vi "Send general mesage.vi"(4 "Content":variant, 6 "Topic":variant, 7 "Sender":string, 8 "error in (no error)":errorcluster, 9 "Recipient":string, 10 "Message":T1={"Sender"="", "Recipient"="", "Topic"=variant(string ""), "Content"=variant, "Time Stamp"=timestamp(0 s since 1904-01-01)} {"Time Stamp" format="%<%H:%M:%S\n%Y/%m/%d>T"}, 11 "Mailbox ref in":T2) -> (0 "error out":errorcluster, 2 "timed out?":bool, 3 "mailbox ref out":T2)   [LabVIEW 2021, in "MatS Libs.lvlib"]
doc: "Puts general message into mailbox. If any information is missing, it is autofilled with default value.\nDefault values:\nIf optional imputs are not empty, they obverwrites message cluster."
uses:
  <userlib>/MatS Libs/MatS Mailman/TypeDefs/Mailbox ref.ctl
  <userlib>/MatS Libs/MatS Mailman/TypeDefs/General message.ctl
  <userlib>/MatS Libs/MatS Libs.lvlib
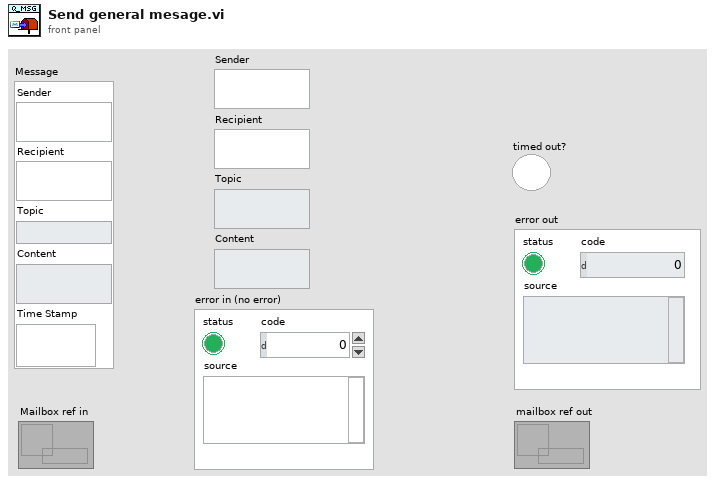
[diagram p1: front panel]
types:
  T1 = typedef "MatS Libs.lvlib/General message.ctl" = cluster{"Sender":string, "Recipient":string, "Topic":variant, "Content":variant, "Time Stamp":timestamp}
  T2 = typedef "MatS Libs.lvlib/Mailbox ref.ctl" = refnum<queue>
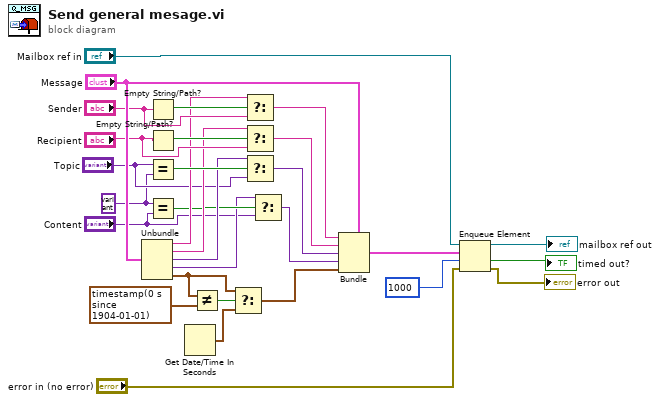
[diagram p0: block diagram]
diagram:
  w1 = variant ("y")
  n1 = Unbundle("Message") -> ("Sender"=w12:string, "Recipient"=w11:string, "Topic"=w10:variant, "Content"=w8:variant, "Time Stamp"=w23:timestamp)
  n2 = Empty String/Path?(string/path="Sender") -> (empty?=w17:bool)
  n3 = Empty String/Path?(string/path="Recipient") -> (empty?=w14:bool)
  n4 = Equal?(x="Topic", y=w1) -> (x = y?=w15:bool)
  n5 = Equal?(x=w1, y="Content") -> (x = y?=w9:bool)
  n6 = Get Date/Time In Seconds() -> (seconds since 1Jan1904=w22:timestamp)
  n7 = Not Equal?(x=w23, y=timestamp(0 s since 1904-01-01) ("Time Stamp")) -> (x != y?=w24:bool)
  n8 = Select(t=w23, s=w24, f=w22) -> (s? t:f=w20:timestamp)
  n9 = Select(t=w12, s=w17, f="Sender") -> (s? t:f=w4:string)
  n10 = Select(t=w11, s=w14, f="Recipient") -> (s? t:f=w3:string)
  n11 = Select(t=w10, s=w15, f="Topic") -> (s? t:f=w5:variant)
  n12 = Select(t=w8, s=w9, f="Content") -> (s? t:f=w6:variant)
  n13 = Bundle(cluster="Message", "Sender"=w4, "Recipient"=w3, "Topic"=w5, "Content"=w6, "Time Stamp"=w20) -> (w21:T1)
  n14 = Enqueue Element(queue="Mailbox ref in", element=w21, timeout in ms (-1)=1000, error in (no error)="error in (no error)") -> (queue out=→"mailbox ref out":T2, timed out?=→"timed out?":bool, error out=→"error out":errorcluster)
